vi "Get Master Base DIR.vi"(4 "error in (no error)":errorcluster, 6 "relative path":string) -> (0 "error out":errorcluster, 2 "Master DIR":string)   [LabVIEW 2020, in "TALOS.lvlib" / "Kasli Wrapper 2.0.lvlib" / "Kasli Wrapper 2.0.lvclass"]
uses:
  Kasli Wrapper 2.0.lvclass
  Kasli/Kasli.lvclass
  Kasli Wrapper 2.0.lvlib
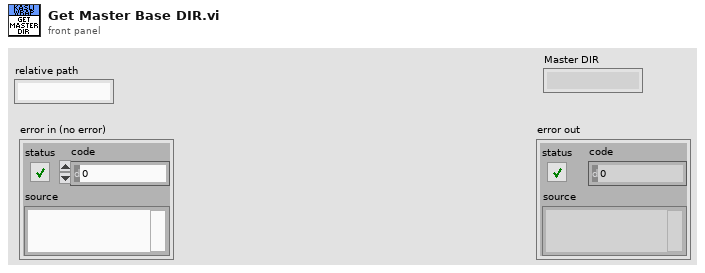
[diagram p1: front panel]
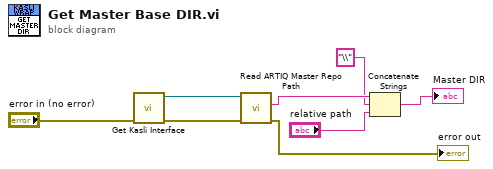
[diagram p0: block diagram]
diagram:
  n1 = call "Get Kasli Interface.vi"("error in"="error in (no error)") -> ("error out"=w1:errorcluster, "Kasli Interface"=w2:refnum<class "Kasli.lvclass">)  [unwired: 9 in]
  n2 = call-dynamic "Read ARTIQ Master Repo Path.vi"("error in (no error)"=w1, "Kasli in"=w2) -> ("error out"=→"error out":errorcluster, "ARTIQ Master Repo Path"=w8:string)  [unwired: 7 in, 1 out]
  n3 = Concatenate Strings(w8, "\\" ("string"), "relative path") -> (→"Master DIR":string)
